vi "Search.vi"(8 "error in (no error)":errorcluster, 9 "SearchMethod":T1, 11 "Tree in":refnum<class "Tree.lvclass">) -> (0 "error out":errorcluster, 1 "found":bool, 2 "Node":refnum<data-value>, 3 "Tree out":refnum<class "Tree.lvclass">)   [LabVIEW 2014, in "Tree.lvlib" / "Tree.lvclass"]
doc: "Searches the tree based on method choosen."
uses:
  <userlib>/AdvancedDataStructures/ClassBased/Tree/Tree.lvclass
  <userlib>/AdvancedDataStructures/ClassBased/TreeNode/TreeNode.lvclass
  <userlib>/AdvancedDataStructures/ClassBased/Tree/SearchMethod.ctl
  <userlib>/AdvancedDataStructures/ClassBased/Tree/Tree.lvclass/Tree.ctl
  <userlib>/AdvancedDataStructures/ClassBased/LinkedList/LinkedList.lvclass
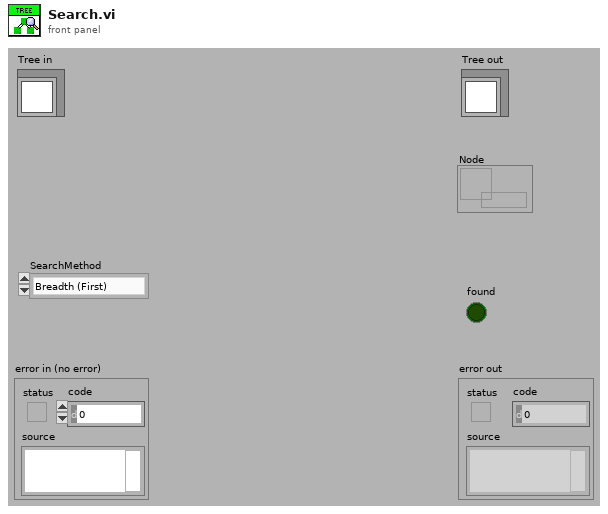
[diagram p1: front panel]
types:
  T1 = typedef "Tree.lvlib/Tree.lvclass/SearchMethod.ctl" = enum16{"Breadth (First)", "Depth (First)", "Best First", "Breadth (Exhaustive)", "Depth (Exhaustive)"}
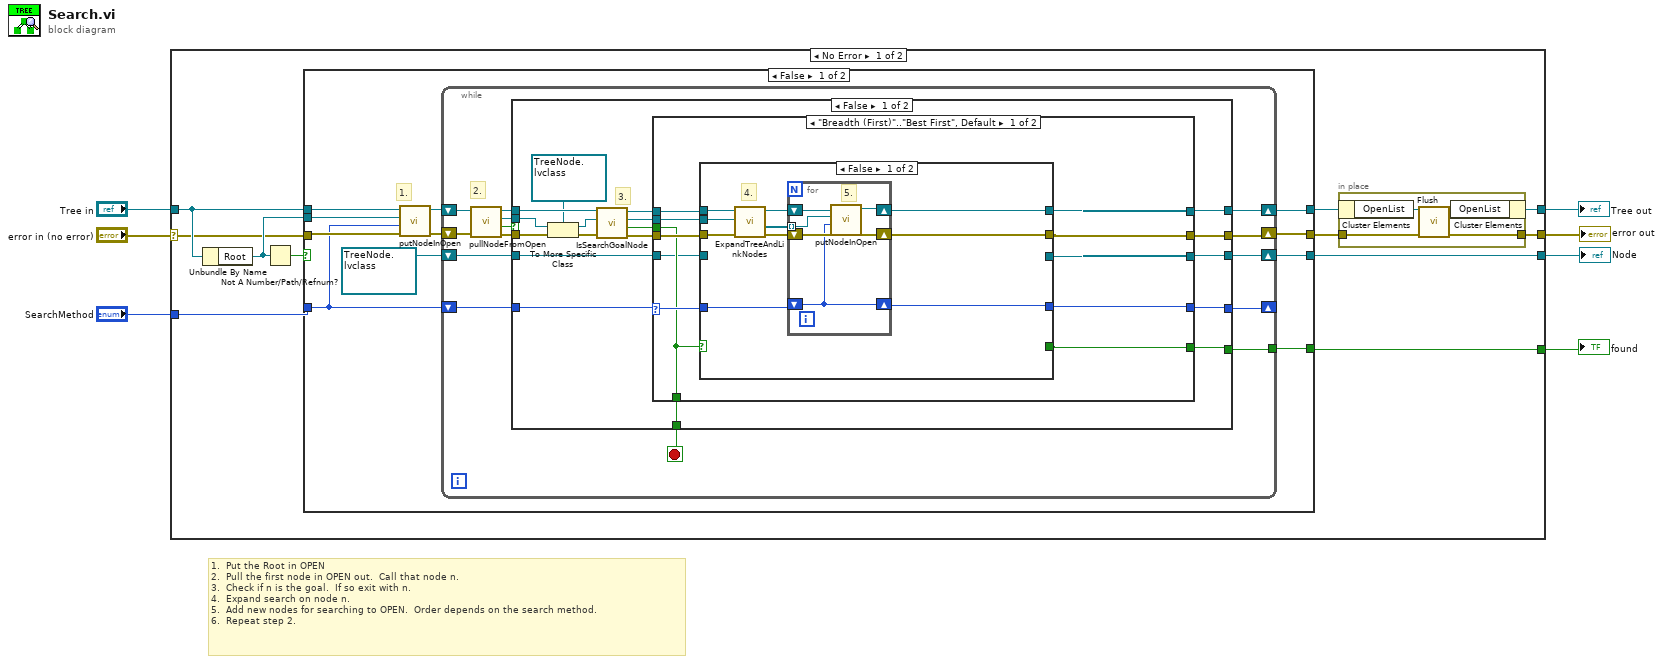
[diagram p0: block diagram]
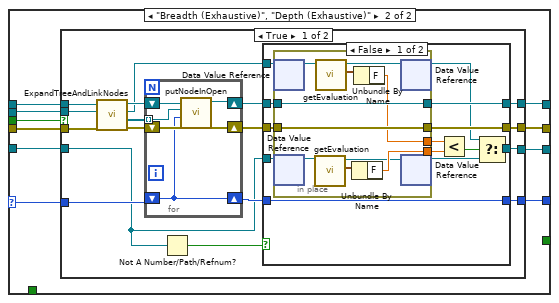
[diagram p3: hidden frame]
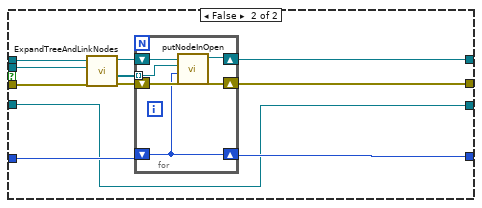
[diagram p5: hidden frame]
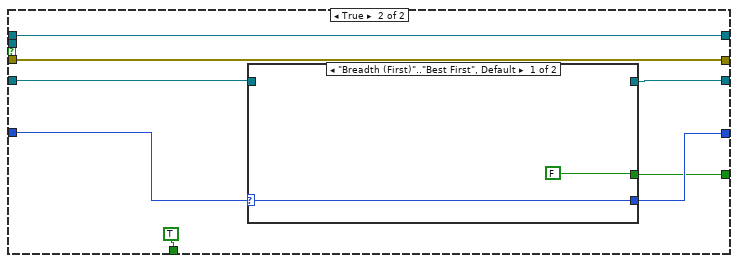
[diagram p6: hidden frame]
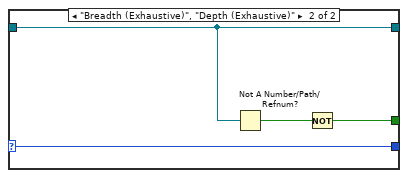
[diagram p7: hidden frame]
diagram:
  # "1.  Put the Root in OPEN\n2.  Pull the first node in OPEN out.  Call that node n.\n3.  Check if n is the goal.  If so exit with n.\n4.  Expand search on node n.\n5.  Add new nodes for searching to OPEN.  Order depends on the search method.\n6.  Repeat step 2."
  n1 = case shown="No Error" "error in (no error)" {
    selector: "error in (no error)" -> [w15 w192]
    tunnel: [w10 w192] -> w6
    tunnel: [w8 w191] -> w4
    tunnel: "Tree in" -> [w17 w191]
    tunnel: [w14 _] -> w3
    tunnel: "SearchMethod" -> [w13 _]
    tunnel: [w12 _] -> w1
    frame No Error {
      n2 = Unbundle By Name(w17) -> ("Root"=w16:refnum<data-value>)
      n3 = Not A Number/Path/Refnum?(number/path/refnum=w16) -> (NaN/Path/Refnum?=w18:bool)
      n4 = case shown="False" w18 {
        tunnel: w17 -> [w33 w189]
        tunnel: w16 -> [w31 _]
        tunnel: w15 -> [w30 w190]
        tunnel: [w27 w189] -> w9
        tunnel: [w26 w190] -> w11
        tunnel: [w28 _] -> w14
        tunnel: w13 -> [w24 _]
        tunnel: [w25 _] -> w12
        frame False {
          # "1."
          n5 = call <userlib>:"putNodeInOpen.vi"("error in (no error)"=w30, "SearchMethod"=w24, "TreeNode"=w31, "Tree in"=w33) -> ("error out"=w29:errorcluster, "Tree out"=w32:refnum<class "Tree.lvclass">)  [unwired: 6 in]
          n6 = while {
            shift-right: [w40] -> w27
            shift-left: w32 -> [w46]
            shift-right: [w39] -> w26
            shift-left: w29 -> [w47]
            tunnel: [w41] -> w28
            shift-right: [w36] -> _
            shift-left: w24 -> [w37]
            shift-right: [w38] -> w25
            shift-left: refnum<data-value> refnum ("NodeToIdentify out") -> [w34]
            stop <- w44 stop-if-true
            # "2."
            n7 = call <userlib>:"pullNodeFromOpen.vi"("error in (no error)"=w47, "Tree in"=w46) -> ("error out"=w45:errorcluster, "empty"=w43:bool, "RemovedNode"=w35:refnum<data-value>, "Tree out"=w42:refnum<class "Tree.lvclass">)  [unwired: 6 in]
            n8 = case shown="False" w43 {
              tunnel: w45 -> [w62 w180]
              tunnel: [w56 TRUE ("found")] -> w44
              tunnel: w42 -> [w65 w181]
              tunnel: [w48 w177] -> w41
              tunnel: [w50 w181] -> w40
              tunnel: [w51 w180] -> w39
              tunnel: [w49 w175] -> w38
              tunnel: w37 -> [w59 w179]
              tunnel: [w52 w178] -> w36
              tunnel: w35 -> [w63 _]
              tunnel: w34 -> [w58 w176]
              frame False {
                # "3."
                n9 = To More Specific Class(target class=refnum<data-value> refnum ("Node"), reference=w63, error in=w62) -> (specific class reference=w60:refnum<data-value>, error out=w61:errorcluster)
                n10 = call-dynamic "IsSearchGoalNode.vi"("error in (no error)"=w61, "PossibleSearchGoal in"=w60, "Tree in"=w65) -> ("error out"=w55:errorcluster, "IsNode"=w57:bool, "PossibleSearchGoal out"=w54:refnum<data-value>, "Tree out"=w53:refnum<class "Tree.lvclass">)  [unwired: 5 in]
                n11 = case shown="\"Breadth (First)\"..\"Best First\", Default" w59 {
                  selector: w59 -> [w76 w106]
                  tunnel: [w71 w104] -> w52
                  tunnel: w58 -> [w67 w99]
                  tunnel: w57 -> [w68 w102]
                  tunnel: [w68 _] -> w56
                  tunnel: [w69 w98] -> w49
                  tunnel: w55 -> [w72 w103]
                  tunnel: w54 -> [w73 w105]
                  tunnel: w53 -> [w75 w107]
                  tunnel: [w74 w101] -> w50
                  tunnel: [w70 w100] -> w51
                  tunnel: [w66 _] -> w48
                  frame "Breadth (First)".."Best First", Default {
                    n12 = case shown="False" w68 {
                      selector: w68 -> [_ w97]
                      tunnel: [_ w97] -> w66
                      tunnel: w75 -> [w83 w96]
                      tunnel: [w85 w96] -> w74
                      tunnel: [w84 w94] -> w70
                      tunnel: w73 -> [w79 w93]
                      tunnel: w76 -> [w86 w95]
                      tunnel: [w78 w95] -> w71
                      tunnel: w72 -> [w77 w94]
                      tunnel: [_ w93] -> w69
                      tunnel: w67 -> [_ _]
                      frame False {
                        # "4."
                        n13 = call <userlib>:"ExpandTreeAndLinkNodes.vi"("error in (no error)"=w77, "ToExpand in"=w79, "Tree in"=w83) -> ("error out"=w81:errorcluster, "ExpandedSearchNodes"=w80:refnum<data-value>[], "Tree out"=w82:refnum<class "Tree.lvclass">)  [unwired: 5 in, 1 out]
                        n14 = for {
                          shift-right: [w90] -> w85
                          shift-left: w82 -> [w92]
                          tunnel: w80 -> [w91] mode=indexing
                          shift-right: [w88] -> w84
                          shift-left: w81 -> [w89]
                          shift-right: [w87] -> w78
                          shift-left: w86 -> [w87]
                          # "5."
                          n15 = call <userlib>:"putNodeInOpen.vi"("error in (no error)"=w89, "SearchMethod"=w87, "TreeNode"=w91, "Tree in"=w92) -> ("error out"=w88:errorcluster, "Tree out"=w90:refnum<class "Tree.lvclass">)  [unwired: 6 in]
                        }
                      }
                      frame True {
                      }
                    }
                  }
                  frame "Breadth (Exhaustive)", "Depth (Exhaustive)" {
                    n16 = case shown="True" w102 {
                      tunnel: w107 -> [w121 w165]
                      tunnel: w106 -> [w120 w164]
                      tunnel: w105 -> [w119 w163]
                      tunnel: [w109 w162] -> w104
                      tunnel: w103 -> [w118 w161]
                      tunnel: [w114 w160] -> w101
                      tunnel: [w113 w159] -> w100
                      tunnel: w99 -> [w108 w158]
                      tunnel: [w112 w158] -> w98
                      frame True {
                        n17 = call <userlib>:"ExpandTreeAndLinkNodes.vi"("error in (no error)"=w118, "ToExpand in"=w119, "Tree in"=w121) -> ("error out"=w123:errorcluster, "ExpandedSearchNodes"=w122:refnum<data-value>[], "ToExpand out"=w117:refnum<data-value>, "Tree out"=w124:refnum<class "Tree.lvclass">)  [unwired: 5 in]
                        n18 = for {
                          shift-right: [w155] -> w115
                          shift-left: w124 -> [w157]
                          tunnel: w122 -> [w156] mode=indexing
                          shift-right: [w153] -> w116
                          shift-left: w123 -> [w154]
                          shift-right: [w152] -> w110
                          shift-left: w120 -> [w152]
                          n19 = call <userlib>:"putNodeInOpen.vi"("error in (no error)"=w154, "SearchMethod"=w152, "TreeNode"=w156, "Tree in"=w157) -> ("error out"=w153:errorcluster, "Tree out"=w155:refnum<class "Tree.lvclass">)  [unwired: 6 in]
                        }
                        n20 = Not A Number/Path/Refnum?(number/path/refnum=w108) -> (NaN/Path/Refnum?=w111:bool)
                        n21 = case shown="False" w111 {
                          tunnel: w117 -> [w137 w148]
                          tunnel: w116 -> [w136 w150]
                          tunnel: w115 -> [w135 w151]
                          tunnel: [w134 w151] -> w114
                          tunnel: [w133 w150] -> w113
                          tunnel: [w127 w148] -> w112
                          tunnel: w110 -> [w126 w149]
                          tunnel: [w126 w149] -> w109
                          tunnel: w108 -> [w125 _]
                          frame False {
                            n22 = in-place {
                              in-place-border: w136 -> [w147]
                              in-place-border: [w147] -> w133
                              in-place-border: w135 -> [w146]
                              in-place-border: [w146] -> w134
                              in-place-border: [w141] -> w132
                              in-place-border: [w139] -> w131
                              n23 = in-place-dvr #1(w137) -> (w144:refnum<class "TreeNode.lvclass">)  [unwired: 1 out]
                              n24 = in-place-dvr #2(w125) -> (w145:refnum<class "TreeNode.lvclass">)  [unwired: 1 out]
                              n25 = call <userlib>:"getEvaluation.vi"("TreeNode in"=w145) -> ("evaluation"=w140:cluster{"F":dbl, "G":dbl, "H":dbl}, "TreeNode out"=w138:refnum<class "TreeNode.lvclass">)  [unwired: 8 in, 1 out]
                              n26 = call <userlib>:"getEvaluation.vi"("TreeNode in"=w144) -> ("evaluation"=w142:cluster{"F":dbl, "G":dbl, "H":dbl}, "TreeNode out"=w143:refnum<class "TreeNode.lvclass">)  [unwired: 8 in, 1 out]
                              n27 = Unbundle By Name(w140) -> ("F"=w139:dbl)
                              n28 = Unbundle By Name(w142) -> ("F"=w141:dbl)
                              n29 = in-place-dvr #1(w143) -> (w129:refnum<data-value>)  [unwired: 1 out]
                              n30 = in-place-dvr #2(w138) -> (w128:refnum<data-value>)  [unwired: 1 out]
                            }
                            n31 = Less?(x=w132, y=w131) -> (x < y?=w130:bool)
                            n32 = Select(t=w129, s=w130, f=w128) -> (s? t:f=w127:refnum<data-value>)
                          }
                          frame True {
                          }
                        }
                      }
                      frame False {
                        n33 = call <userlib>:"ExpandTreeAndLinkNodes.vi"("error in (no error)"=w161, "ToExpand in"=w163, "Tree in"=w165) -> ("error out"=w167:errorcluster, "ExpandedSearchNodes"=w166:refnum<data-value>[], "Tree out"=w168:refnum<class "Tree.lvclass">)  [unwired: 5 in, 1 out]
                        n34 = for {
                          shift-right: [w172] -> w160
                          shift-left: w168 -> [w174]
                          tunnel: w166 -> [w173] mode=indexing
                          shift-right: [w170] -> w159
                          shift-left: w167 -> [w171]
                          shift-right: [w169] -> w162
                          shift-left: w164 -> [w169]
                          n35 = call <userlib>:"putNodeInOpen.vi"("error in (no error)"=w171, "SearchMethod"=w169, "TreeNode"=w173, "Tree in"=w174) -> ("error out"=w170:errorcluster, "Tree out"=w172:refnum<class "Tree.lvclass">)  [unwired: 6 in]
                        }
                      }
                    }
                  }
                }
              }
              frame True {
                n36 = case shown="\"Breadth (First)\"..\"Best First\", Default" w179 {
                  selector: w179 -> [w184 w188]
                  tunnel: [w184 w188] -> w178
                  tunnel: [FALSE w185] -> w177
                  tunnel: w176 -> [_ w187]
                  tunnel: [_ w187] -> w175
                  frame "Breadth (First)".."Best First", Default {
                  }
                  frame "Breadth (Exhaustive)", "Depth (Exhaustive)" {
                    n37 = Not A Number/Path/Refnum?(number/path/refnum=w187) -> (NaN/Path/Refnum?=w186:bool)
                    n38 = Not(x=w186) -> (.not. x?=w185:bool)
                  }
                }
              }
            }
          }
        }
        frame True {
          # "No nodes in tree.  Cannot be found."
        }
      }
      n39 = in-place {
        in-place-border: w11 -> [w22]
        in-place-border: [w21] -> w10
        n40 = in-place-cluster #3(w9) -> ("OpenList"=w20:refnum<class "BasicSortedList.lvclass">)
        n41 = call <userlib>:"Flush.vi"("error in (no error)"=w22, "LinkedList in"=w20) -> ("error out"=w21:errorcluster, "LinkedList out"=w19:refnum<class "BasicSortedList.lvclass">)  [unwired: 7 in, 1 out]
        n42 = in-place-cluster #3("OpenList"=w19) -> (w8:refnum<class "Tree.lvclass">)
      }
    }
    frame Error {
    }
  }
  "error out" <- w6
  "Tree out" <- w4
  "found" <- w3
  "Node" <- w1
